vi "main.vi"() -> ()   [LabVIEW 2021]
uses:
  <vilib>/Instr/_visa.llb/VISA Configure Serial Port (Instr).vi
panel:
  out "Indicator: Position Feedback (‰)":u16(slide) scale=0.0..1000.0
  out "Pressure Force Feedback (N)":dbl(graph)
  in  "Force limitation (N)":dbl=1.0
  in  "Control: Position Control (‰)":u16(slide) step=1 scale=0.0..1000.0
  in  "STOP":bool
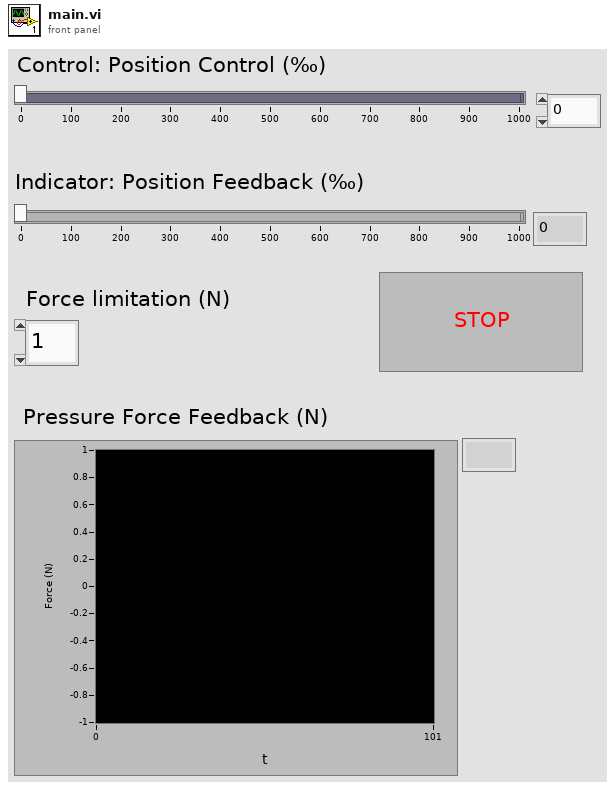
[diagram p1: front panel]
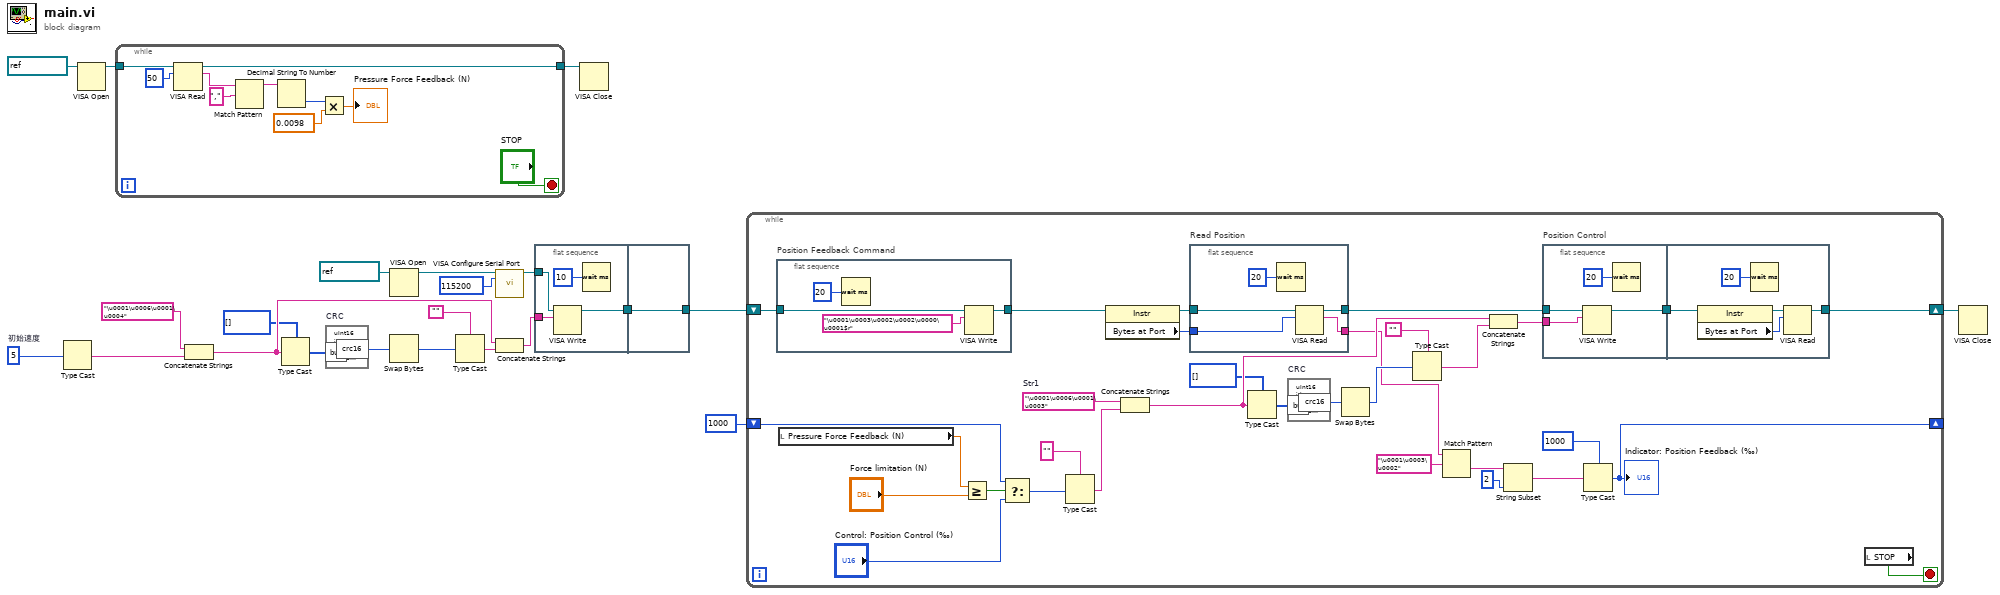
[diagram p0: block diagram]
diagram:
  w6 = u16 5  # 初始速度
  n1 = Type Cast(x=w6) -> (*(type *) &x=w8:string)  [unwired: 1 in]
  n2 = VISA Open(VISA resource name=refnum<visa-resource-name> "COM9" ("VISA资源名称")) -> (VISA resource name=w20:refnum<visa-resource-name>)  [unwired: 4 in, 1 out]
  n3 = while {
    tunnel: w20 -> [w32]
    tunnel: [w31] -> w19
    stop <- "STOP" stop-if-true
    n4 = VISA Read(VISA resource name=w32, byte count=u32 50 ("字节总数")) -> (VISA resource name out=w31:refnum<visa-resource-name>, read buffer=w28:string)  [unwired: 1 in, 2 out]
    n5 = Match Pattern(string=w28, regular expression=",") -> (before substring=w26:string)  [unwired: 1 in, 3 out]
    n6 = Decimal String To Number(string=w26) -> (number=w25:i32)  [unwired: 2 in, 1 out]
    n7 = Multiply(x=w25, y=0.0098) -> (x*y=→"Pressure Force Feedback (N)":dbl)
  }
  n8 = Concatenate Strings("\u0001\u0006\u0001\u0004" ("设置速度"), w8) -> (w10:string)
  n9 = Type Cast(type=u8[] [], x=w10) -> (*(type *) &x=w15:u8[])
  n10 = formula code="uInt16 i,j,crc16,temp;\ncrc16=0xffff;\nfor(i=0;i<sizeOfDim(buf,0);i++)\n{\n    crc16^=buf[i];\n    for(j=0;j<8;j++)\n    {\n      temp=crc16&0x0001;\n      crc16>>=0x01;\n      if(temp) crc16^=0XA001;\n     }\n}" "CRC"("buf"=w15) -> ("crc16"=w14:u16)
  n11 = VISA Open(VISA resource name=refnum<visa-resource-name> "COM6" ("VISA资源名称")) -> (VISA resource name=w3:refnum<visa-resource-name>)  [unwired: 4 in, 1 out]
  n12 = Swap Bytes(anything=w14) -> (byte swapped=w13:u16)
  n13 = Type Cast(type="", x=w13) -> (*(type *) &x=w11:string)
  n14 = call-poly "VISA Configure Serial Port"("VISA resource name"=w3, "baud rate (9600)"=u32 115200) -> ("VISA resource name out"=w1:refnum<visa-resource-name>)  [unwired: 12 in, 1 out]
  n15 = Concatenate Strings(w10, w11) -> (w5:string)
  n16 = flat-sequence {
    tunnel: w1 -> [w36]
    tunnel: w5 -> [w35]
    tunnel: [w33] -> w2
    tunnel: [w37] -> w17
    tunnel: w2 -> [w37]
    frame #0 {
      n17 = VISA Write ("VISA写入")(VISA resource name=w36, write buffer=w35) -> (VISA resource name out=w33:refnum<visa-resource-name>)  [unwired: 1 in, 2 out]
      n18 = Wait (ms)(milliseconds to wait=u32 10 ("等待时间（毫秒）")) -> ()  [unwired: 1 out]
    }
    frame #1 {
    }
  }
  n19 = VISA Close(VISA resource name=w19) -> ()  [unwired: 1 in, 1 out]
  n20 = while {
    shift-right: [w40] -> _
    shift-left: u16 1000 ("Position Control (‰) 2") -> [w54]
    shift-right: [w39] -> w16
    shift-left: w17 -> [w51]
    stop <- w69 stop-if-true
    w68 = "\u0001\u0006\u0001\u0003"  # Str1
    n21 = flat-sequence "Position Feedback Command" {
      tunnel: w51 -> [w86]
      tunnel: [w85] -> w50
      frame #0 {
        n22 = Wait (ms)(milliseconds to wait=u32 20 ("等待时间（毫秒）")) -> ()  [unwired: 1 out]
        n23 = VISA Write ("VISA写入")(VISA resource name=w86, write buffer="\u0001\u0003\u0002\u0002\u0000\u0001$r" ("设置速度")) -> (VISA resource name out=w85:refnum<visa-resource-name>)  [unwired: 1 in, 2 out]
      }
    }
    n24 = local read "Pressure Force Feedback (N)"() -> (w59:dbl)
    n25 = Greater Or Equal?(x=w59, y="Force limitation (N)") -> (x >= y?=w55:bool)
    n26 = Select(t=w54, s=w55, f="Control: Position Control (‰)") -> (s? t:f=w53:u16)
    n27 = Type Cast(type="" ("类型"), x=w53) -> (*(type *) &x=w67:string)
    n28 = property class="Instr"(reference=w50) -> (reference out=w49:refnum<visa-resource-name>, "Bytes at Port"=w47:u32)  [unwired: 1 in, 1 out]
    n29 = Concatenate Strings(w68, w67) -> (w62:string)
    n30 = flat-sequence "Read Position" {
      tunnel: w49 -> [w83]
      tunnel: [w82] -> w48
      tunnel: w47 -> [w81]
      tunnel: [w80] -> w46
      frame #0 {
        n31 = Wait (ms)(milliseconds to wait=u32 20 ("等待时间（毫秒）")) -> ()  [unwired: 1 out]
        n32 = VISA Read(VISA resource name=w83, byte count=w81) -> (VISA resource name out=w82:refnum<visa-resource-name>, read buffer=w80:string)  [unwired: 1 in, 2 out]
      }
    }
    n33 = Type Cast(type=u8[] [], x=w62) -> (*(type *) &x=w66:u8[])
    n34 = formula code="uInt16 i,j,crc16,temp;\ncrc16=0xffff;\nfor(i=0;i<sizeOfDim(buf,0);i++)\n{\n    crc16^=buf[i];\n    for(j=0;j<8;j++)\n    {\n      temp=crc16&0x0001;\n      crc16>>=0x01;\n      if(temp) crc16^=0XA001;\n     }\n}" "CRC"("buf"=w66) -> ("crc16"=w65:u16)
    n35 = Swap Bytes(anything=w65) -> (byte swapped=w64:u16)
    n36 = Type Cast(type="", x=w64) -> (*(type *) &x=w61:string)
    n37 = Match Pattern(string=w46, regular expression="\u0001\u0003\u0002" ("设置速度")) -> (after substring=w44:string)  [unwired: 1 in, 3 out]
    n38 = Concatenate Strings(w62, w61) -> (w56:string)
    n39 = String Subset(string=w44, length (rest)=2 ("长度（剩余）")) -> (substring=w42:string)  [unwired: 1 in]
    n40 = flat-sequence "Position Control" {
      tunnel: w56 -> [w73]
      tunnel: w48 -> [w71]
      tunnel: [w72] -> w38
      tunnel: [w75] -> w39
      tunnel: w38 -> [w78]
      frame #0 {
        n41 = VISA Write(VISA resource name=w71, write buffer=w73) -> (VISA resource name out=w72:refnum<visa-resource-name>)  [unwired: 1 in, 2 out]
        n42 = Wait (ms)(milliseconds to wait=u32 20 ("等待时间（毫秒）")) -> ()  [unwired: 1 out]
      }
      frame #1 {
        n43 = property class="Instr"(reference=w78) -> (reference out=w77:refnum<visa-resource-name>, "Bytes at Port"=w76:u32)  [unwired: 1 in, 1 out]
        n44 = Wait (ms)(milliseconds to wait=u32 20 ("等待时间（毫秒）")) -> ()  [unwired: 1 out]
        n45 = VISA Read(VISA resource name=w77, byte count=w76) -> (VISA resource name out=w75:refnum<visa-resource-name>)  [unwired: 1 in, 3 out]
      }
    }
    n46 = Type Cast(type=u16 1000 ("Position Control (‰) 2"), x=w42) -> (*(type *) &x=w40:u16)
    "Indicator: Position Feedback (‰)" <- w40
    n47 = local read "STOP"() -> (w69:bool)
  }
  n48 = VISA Close(VISA resource name=w16) -> ()  [unwired: 1 in, 1 out]
